vi "Show Diagram.vi"(8 "error in (no error)":errorcluster) -> (0 "error out":errorcluster)   [LabVIEW 2017, in "FingerPrintMânager.lvlib"]
doc: "This VI tells the Module to show its block diagram to facilitate troubleshooting (add probes, breakpoints, highlight execution, etc).\n\n_____\nBased on Delacor QMH Project Template 4.1.0.59."
uses:
  Show Diagram Argument--cluster.ctl
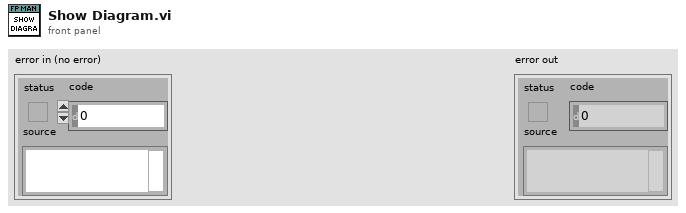
[diagram p1: front panel]
types:
  T1 = typedef "FingerPrintMânager.lvlib/Show Diagram Argument--cluster.ctl" = cluster{"Debug?":bool}
  T2 = typedef "FingerPrintMânager.lvlib/Request Events--cluster.ctl" = cluster{"Stop Module":refnum<user-event>, "Show Panel":refnum<user-event>, "Hide Panel":refnum<user-event>, "Get Module Execution Status":refnum<user-event>, "Show Diagram":refnum<user-event>, "Init":refnum<user-event>, "UnInit":refnum<user-event>, "Write":refnum<user-event>, "Read":refnum<user-event>, "UpdatePump":refnum<user-event>, "StopPump":refnum<user-event>}
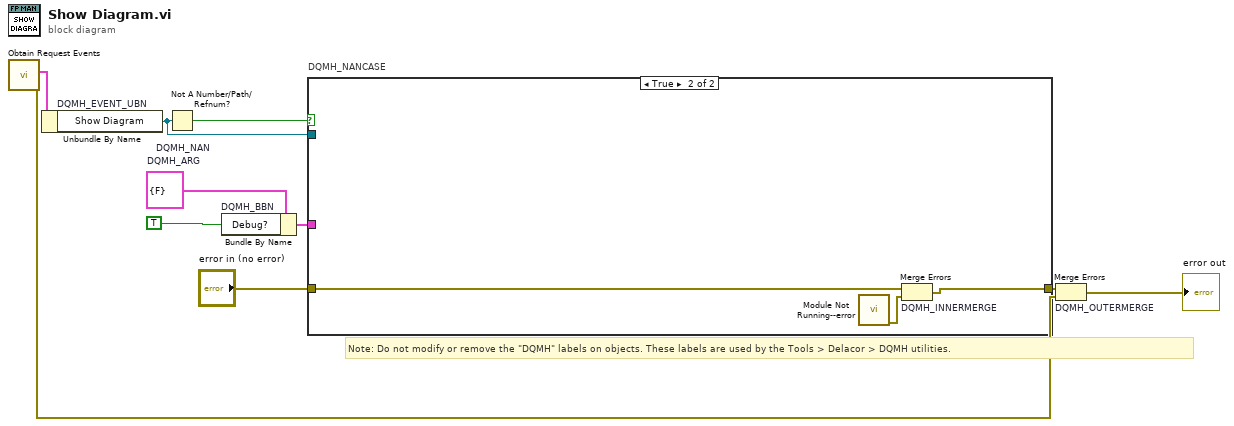
[diagram p0: block diagram]
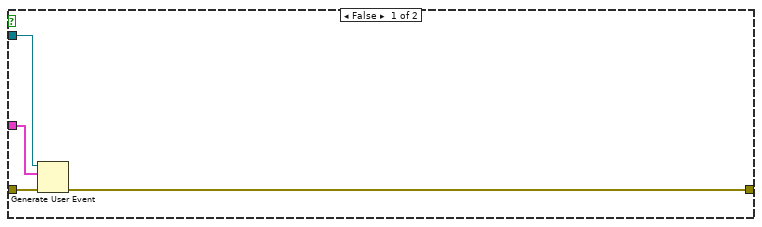
[diagram p2: hidden frame]
diagram:
  w5 = T1 {"Debug?"=FALSE}  # DQMH_ARG
  # "Note: Do not modify or remove the \"DQMH\" labels on objects. These labels are used by the Tools > Delacor > DQMH utilities."
  n1 = call "Obtain Request Events.vi"() -> ("error out"=w1:errorcluster, "FingerPrintMânager Request Events"=w3:T2)  [unwired: 10 in]
  n2 = Unbundle By Name "DQMH_EVENT_UBN"(w3) -> ("Show Diagram"=w6:refnum<user-event>)
  n3 = Not A Number/Path/Refnum? "DQMH_NAN"(number/path/refnum=w6) -> (NaN/Path/Refnum?=w7:bool)
  n4 = Bundle By Name "DQMH_BBN"(cluster=w5, "Debug?"=TRUE) -> (w8:T1)
  n5 = case "DQMH_NANCASE" shown="True" w7 {
    tunnel: "error in (no error)" -> [w14 w17]
    tunnel: [w13 w16] -> w2
    tunnel: w6 -> [w12 _]
    tunnel: w8 -> [w11 _]
    frame False {
      n6 = Generate User Event(user event=w12, event data cluster=w11, error in=w14) -> (error out=w13:errorcluster)  [unwired: 1 in, 1 out]
    }
    frame True {
      n7 = call "Module Not Running--error.vi"() -> ("error out"=w15:errorcluster)  [unwired: 11 in]
      n8 = Merge Errors "DQMH_INNERMERGE"(w17, w15) -> (w16:errorcluster)
    }
  }
  n9 = Merge Errors "DQMH_OUTERMERGE"(w2, w1) -> (→"error out":errorcluster)
